vi "读取表格单元格值.vi"(8 "错误输入（无错误）":errorcluster, 10 "行列":cluster{"行":i32, "列":i32}, 11 "引用输入":refnum<vi>) -> (0 "错误输出":errorcluster, 2 "元素":string, 3 "引用输出":refnum<vi>)   [LabVIEW 2014, in "表格.lvlib"]
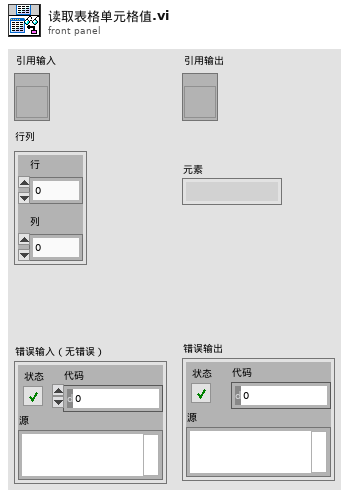
[diagram p1: front panel]
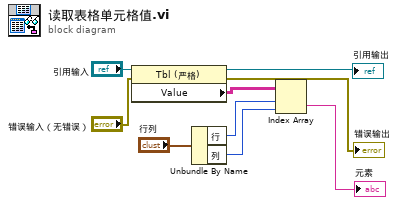
[diagram p0: block diagram]
diagram:
  n1 = property class="Tbl (严格)"(reference="引用输入", error in="错误输入（无错误）") -> (reference out=→"引用输出":refnum<vi>, error out=→"错误输出":errorcluster, "Value"=w9:string[][])
  n2 = Unbundle By Name("行列") -> ("行"=w7:i32, "列"=w6:i32)
  n3 = Index Array(array=w9, index (row)=w7, index (col)=w6) -> (element=→"元素":string)
